vi "Write AI Channels.vi"(8 "error in (no error)":errorcluster, 10 "AI Channels":T1 {"reference index" min=1; "References" items=["", "1", "2", "3"]; "Channel" min=1}, 11 "DSP in":refnum<class "DSP.lvclass">) -> (0 "error out":errorcluster, 3 "DSP out":refnum<class "DSP.lvclass">)   [LabVIEW 2020, in "DSP.lvclass"]
uses:
  DSP.lvclass
  Typedefs/AI.Channel--Cluster--Array.ctl
  Typedefs/AI.Channel--Cluster.ctl
  DSP.lvclass/DSP.ctl
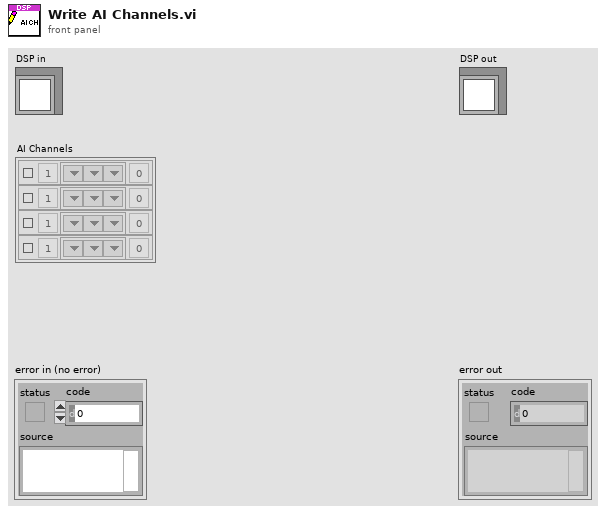
[diagram p1: front panel]
types:
  T1 = typedef "DSP.lvclass/AI.Channel--Cluster--Array.ctl" = T2[]
  T2 = typedef "DSP.lvclass/AI.Channel--Cluster.ctl" = cluster{"Enable?":bool, "Channel":i32, "References":i32[], "reference index":i32}
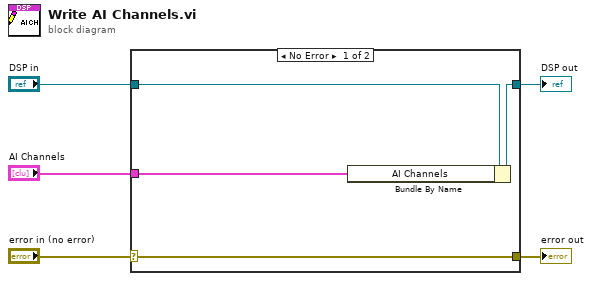
[diagram p0: block diagram]
diagram:
  n1 = case shown="No Error" "error in (no error)" {
    selector: "error in (no error)" -> [w9 w10]
    tunnel: [w9 w10] -> w4
    tunnel: [w7 w11] -> w2
    tunnel: "DSP in" -> [w8 w11]
    tunnel: "AI Channels" -> [w6 _]
    frame No Error {
      n2 = Bundle By Name(cluster=w8, "AI Channels"=w6) -> (w7:refnum<class "DSP.lvclass">)
    }
    frame Error {
    }
  }
  "error out" <- w4
  "DSP out" <- w2
